vi "Dashboard Main.vi"() -> ()   [LabVIEW 2017]
uses:
  <vilib>/Utility/miscctls.llb/LVRowAndColumnTypeDef.ctl
  <vilib>/event_ctls.llb/eventvkey.ctl
  <vilib>/Rock Robotics/Network Tables/NT Read Numeric Array.vi
  <vilib>/Rock Robotics/Network Tables/NT Read Boolean.vi
  <vilib>/Rock Robotics/WPI/Dashboard/WPI_DashboardLogging Global.vi
panel:
  in  "Camera Settings Right":T1={"Frame Rate"=30, "Compression"=30, "Size"=1, "DB Camera Config"=FALSE} {"Frame Rate" scale=1.0..30.0; "Compression" scale=100.0..-1.0; "Size" items=["640x480", "320x240", "160x120"]}
  in  "Camera Name Right":string(combo)="No Camera Selection"
  out "Camera Info":cluster{"Mbps LED":bool, "Mbps":dbl, "fps":dbl} {"fps" format="%#.1g"; "Mbps" format="%#.1g"}
  in  "Camera Settings":T1={"Frame Rate"=30, "Compression"=30, "Size"=1, "DB Camera Config"=FALSE} {"Frame Rate" scale=1.0..30.0; "Compression" scale=100.0..-1.0; "Size" items=["640x480", "320x240", "160x120"]}
  in  "TCP":refnum<k5>
  in  "Rec Mode":enum32{"Stop", "Record", "Playback"}(radio)
  out "Robot IP":string
  out "Image Message":string="Timeout in Camera Communications"
  in  "Dashboard Tab":T2(tab)
  in  "Select Auto":string(combo)="Select Autonomous ..."
  out "NT Connection":bool
  out "MotorChart R":cluster{"Numeric":dbl, "Numeric":dbl}(graph)
  out "MotorChart L":cluster{"Numeric":dbl, "Numeric":dbl}(graph)
  out "MotorSliders R":cluster{"MotorSlide1":dbl, "MotorSlide2":dbl} {"MotorSlide2" scale=-1.0..1.0 scale format="%#_2e"; "MotorSlide1" scale=-1.0..1.0 scale format="%#_2e"}
  out "MotorSliders L":cluster{"MotorSlide1":dbl, "MotorSlide2":dbl} {"MotorSlide2" scale=-1.0..1.0 scale format="%#_2e"; "MotorSlide1" scale=-1.0..1.0 scale format="%#_2e"}
  out "Gyro":dbl(knob) scale=0.0..360.0
  out "JS1 Z":dbl(slide) scale=-1.0..1.0 scale format="%#_2e"
  out "JS1 Graph":cluster{"X":dbl, "Y":dbl}[](graph)
  out "JS1 Buttons":T3
  out "JS2 Z":dbl(slide) scale=-1.0..1.0 scale format="%#_2e"
  out "JS2 Graph":cluster{"X":dbl, "Y":dbl}[](graph)
  out "JS2 Buttons":T3
  out "Mode":T4(ring)=enum."Auto Disabled"
  out "Camera Image Right":T5(plugin-control)
  in  "DB/String 9":string
  in  "DB/String 8":string
  in  "DB/String 7":string
  in  "DB/String 6":string
  in  "DB/String 5":string
  in  "DB/String 4":string
  in  "DB/String 3":string
  in  "DB/String 2":string
  in  "DB/String 1":string
  in  "DB/String 0":string
  in  "DB/Slider 0":dbl(slide) scale=0.0..5.0
  in  "DB/Slider 1":dbl(slide) scale=0.0..5.0
  in  "DB/Slider 2":dbl(slide) scale=0.0..5.0
  in  "DB/Slider 3":dbl(slide) scale=0.0..5.0
  out "DB/LED 3":bool
  out "DB/LED 2":bool
  out "DB/LED 1":bool
  out "DB/LED 0":bool
  in  "DB/Button 3":bool
  in  "DB/Button 2":bool
  in  "DB/Button 1":bool
  in  "DB/Button 0":bool caption="New Name"
  out "Claw Right":bool
  out "Claw Left":bool
  out "Elevator Top":bool
  out "Elevator Bottom":bool
  out "Collector Limit Switch":bool
  out "fast":bool
  out "slow":bool
  out "Phase Indicator":string
  in  "Programming Level":dbl(knob) scale=0.0..11.0
  in  "What color are you?":string(combo)
  out "R3":u32(colorbox)
  out "R2":u32(colorbox)
  out "R1":u32(colorbox)
  out "L3":u32(colorbox)
  out "L2":u32(colorbox)
  out "L1":u32(colorbox)
  in  "Test Slider":dbl(slide) scale=0.0..100.0 scale format="%#_3g"
  in  "On/Off":bool caption="Solenoid"
  in  "Test Name":u16(ring) items=["Select the test to run..."]
  in  "Test Tree":string(tree)
  in  "Motor":cluster{"Value":dbl, "Enable":bool} {"Value" scale=-1.0..1.0 scale format="%#_3g"}
  out "Progress":T6 {"Test Progress" scale=0.0..100.0}
  in  "Rev/Fwd":cluster{"Forward":bool, "Reverse":bool}
  in  "Test Ring":u16(ring) items=["Monochrome", "Color"]
  out "Cmd Status":string
  in  "Execute Command":bool
  in  "Command Params":string[][](table)
  in  "Command Selection":i32(listbox)
  in  "CheckList":i32(listbox)
  out "Tree":string(tree)
  out "Camera Image":T5(plugin-control)
  out "Background":bool
  in  "Camera Name":string(combo)="No Camera Selection"
  # "HW"
  # "HW"
  # "Joysticks"
  # "Drive Motors"
  # "Front"
  # "Right"
  # "Left"
  # "Back"
  # "If you need that extra push over the cliff put it to eleven. These go to eleven."
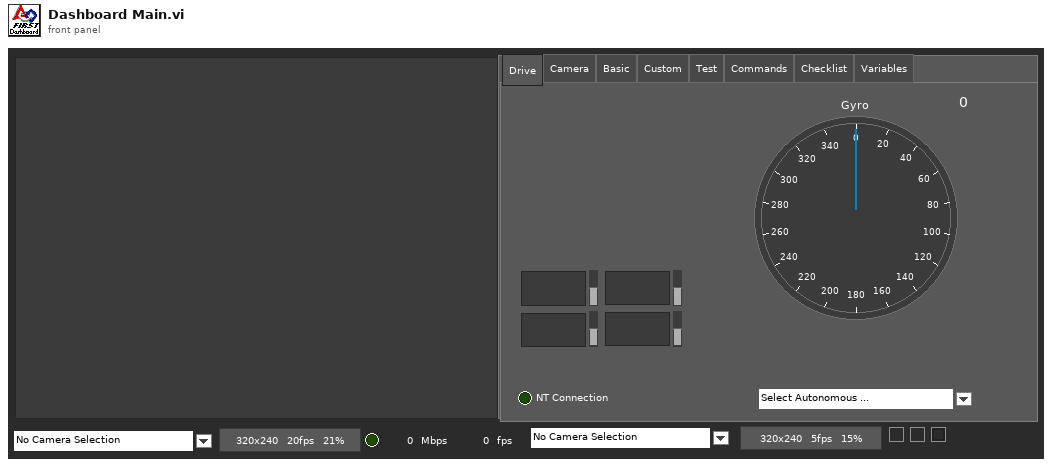
[diagram p1: front panel]
types:
  T1 = cluster{"Frame Rate":i32, "Compression":i32, "Size":u16, "DB Camera Config":bool}
  T2 = enum32{"Drive", "Camera", "Basic", "Custom", "Test", "Commands", "Checklist", "Variables"}
  T3 = cluster{bool, bool, bool, bool, bool, bool, bool, bool, bool, bool, bool, bool}
  T4 = enum8{"Tele-Op Disabled", "Tele-Op Enabled", "Auto Disabled", "Auto Enabled", "Test Disabled", "Test Enabled", "Disconnected", "No Code", "E-Stop"}
  T5 = typedef "IMAQ Image.ctl" = refnum<image>
  T6 = cluster{"Test Progress":u8, "Test Progress Text":string}
  T7 = cluster{"Save Path":path, "Interval (s)":dbl, "Keep":i32}
  T8 = typedef "Image Type" = u32
  T9 = cluster{"IDs":cluster{"RPC field ID":u16, "Unique ID":u16}, "String":string}
  T10 = cluster{"Error Strings":string, "Disable Counts":cluster{u16, u16}, "Rail Faults":cluster{u16, u16, u16}, "Robot IP":string, "DB Mode":u8, "Event Info":cluster{"Name":string, "Type":u8, "Number":u16, "Replay":u8}}
  T11 = cluster{"Storage":cluster{"Disk Free":u64, "RAM Block":u32, "RAM free":u32}, "CPU Utilization":cluster{"CPU % ISR":sgl, "CPU % Time Crit":sgl, "CPU % Timed Str":sgl, "CPU % High":sgl, "CPU % Above":sgl, "CPU % Normal":sgl, "CPU % Low":sgl}, "CAN":cluster{"% Bus Utilization":sgl, "Bus Off Cnt":u32, "TX_FIFO Full Cnt":u32, "Receive Error Cnt":u8, "Transmit Error Cnt":u8}, "HID":cluster{"HID Outputs":u32, "Rumble Low":u16, "Rumble High":u16}[]}
  T12 = cluster{"Status bits":cluster{"Test Mode":bool, "Autonomous":bool, "Enabled":bool, "Code Start":bool, "Brownout":bool, "Reserved 2":bool, "Reserved 3":bool, "E-Stop":bool}, "Code Trace":cluster{"Disabled":bool, "TeleOp":bool, "Auto":bool, "Test":bool}, "Controller Type":enum16{"unknown", "cRIO", "roboRio"}, "Code?":enum16{"unknown", "noCode", "code"}, "Battery V":dbl}
  T13 = cluster{"Control Bits":cluster{"TestMode":bool, "Autonomous":bool, "Enabled":bool, "FMS Present":bool, bool, bool, bool, "E-Stop":bool}, "Team Station ":u8, "Countdown":sgl, "Joystick Values":cluster{"Axes":dbl[], "Buttons":bool[], "POVs":i16[]}[]}
  T14 = cluster{"Axes":dbl[], "Buttons":bool[], "POVs":i16[]}[]
  T15 = cluster{"Axes":dbl[], "Buttons":bool[], "POVs":i16[]}
  T16 = cluster{"Buttons[0]":bool, "Buttons[1]":bool, "Buttons[2]":bool, "Buttons[3]":bool, "Buttons[4]":bool, "Buttons[5]":bool, "Buttons[6]":bool, "Buttons[7]":bool, "Buttons[8]":bool, "Buttons[9]":bool, "Buttons[10]":bool, "Buttons[11]":bool}
  T17 = cluster{"Camera Image":refnum<vi>, "Dashboard Tab":refnum<vi>, "Background":refnum<vi>, "Rec Mode":refnum<vi>, "Test Slider":refnum<vi>, "On/Off ":refnum<vi>, "Test Ring":refnum<vi>, "Rev/Fwd":refnum<vi>, "Test Name":refnum<vi>, "Motor":refnum<vi>, "Progress":refnum<vi>, "CheckList":refnum<vi>, "Tree":refnum<vi>, "Test Tree":refnum<vi>, "Command Params":refnum<vi>, "Command Selection":refnum<vi>, "Execute Command":refnum<vi>, "Cmd Status":refnum<vi>, "Camera Settings":refnum<vi>, "Camera Name":refnum<vi>, "Camera Info":refnum<vi>, "Camera Settings Right":refnum<vi>, "Camera Name Right":refnum<vi>, "Camera Image Right":refnum<vi>}
  T18 = cluster{"Camera Name":string, string, "Saved DB Images Info":cluster{"Save Path":path, "Interval (s)":dbl, "Keep":i32}}
  T19 = cluster{"Camera Name Right":string, string, "Saved DB Images Info":cluster{"Save Path":path, "Interval (s)":dbl, "Keep":i32}}
  T20 = cluster{"Operation":enum16{"Update", "Clear"}, "Color Box":u32}[]
  T21 = typedef "eventvkey.ctl" = enum16{"ASCII", "Enter", "Return", "Shift", "Ctrl", "Alt", "Cmd", "Opt", "Caps", "NumLock", "Clear", "Break", "Up", "Down", "Left", "Right", "Insert", "Delete", "Home", "End", "PageUp", "PageDown", "Escape", "Help", "Pause", "ScrollLock", "F1", "F2", "F3", "F4", "F5", "F6", "F7", "F8", "F9", "F10", "F11", "F12", "F13", "F14", "F15", "F16", "F17", "F18", "F19", "F20", "F21", "F22", "F23", "F24", "Play", "VolumeUp", "VolumeDown", "Mute", "Two Byte Char"}
  T22 = cluster{"Image Size":bool, "Image Type":bool, "Pixel Value":bool, "ROI Information":bool, "Zoom Factor":bool}
  T23 = cluster{"Operation":enum16{"Update", "Clear"}, "Color Box":u32}
  T24 = typedef "LVRowAndColumnTypeDef.ctl" = cluster{"Row":i32, "Column":i32}
  T25 = cluster{"Shift":bool, "Ctrl":bool, "Alt":bool, "Cmd":bool, "Opt":bool}
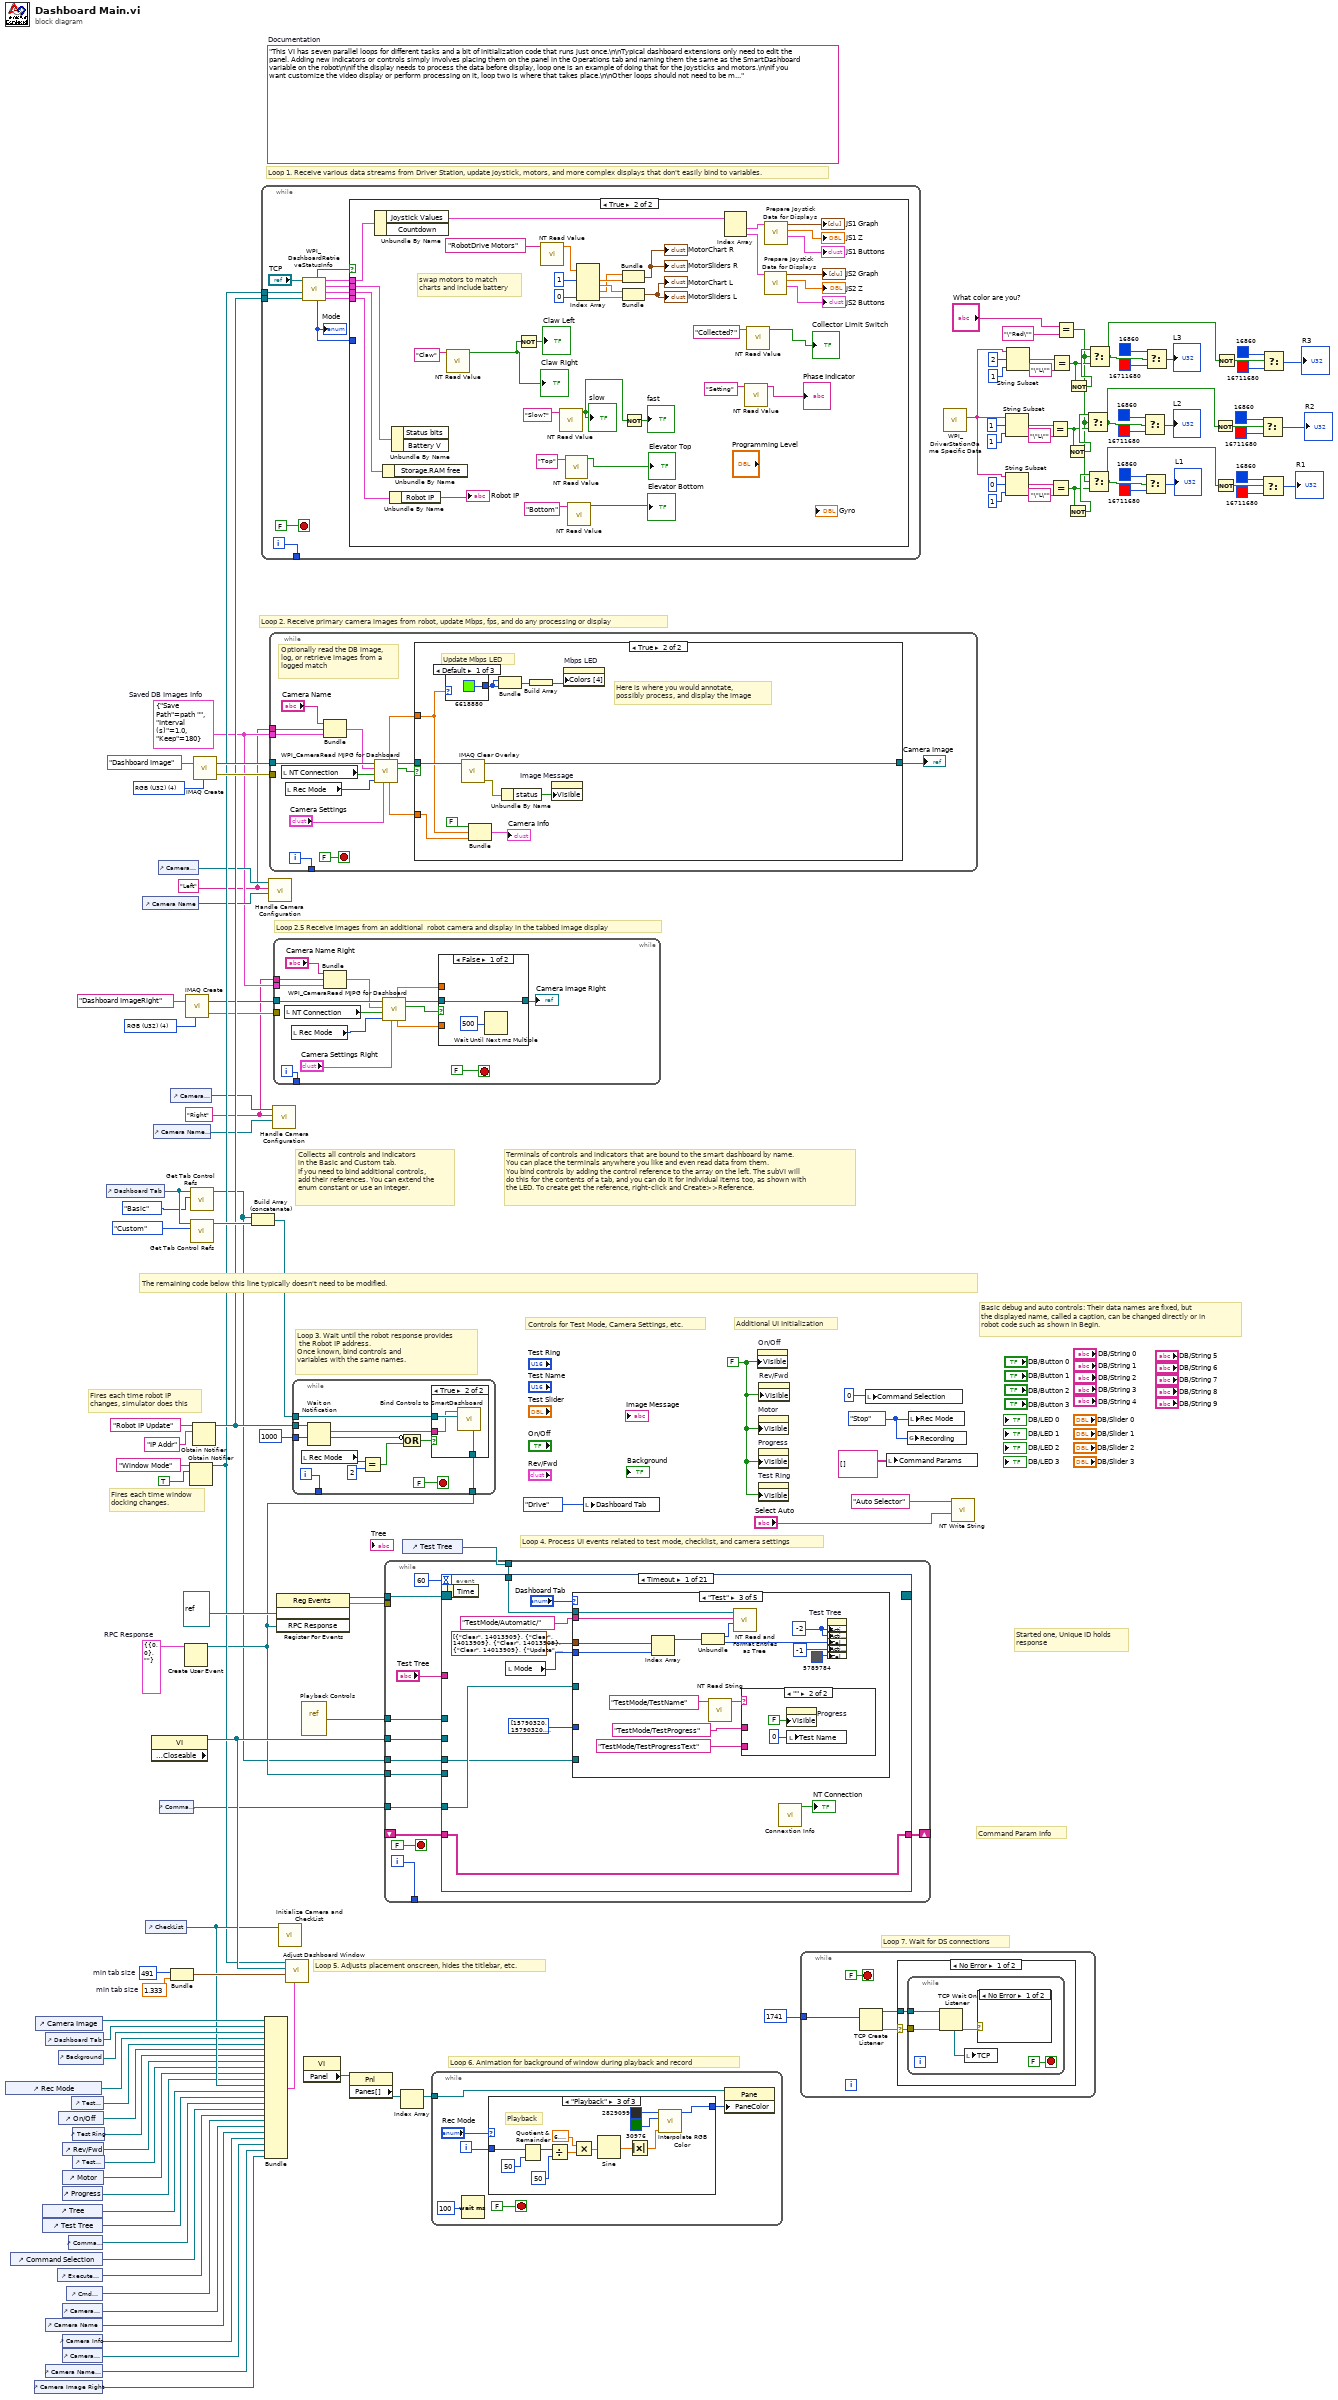
[diagram p0: block diagram]
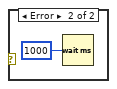
[diagram p3: hidden frame]
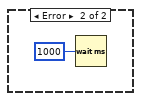
[diagram p4: hidden frame]
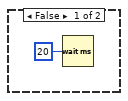
[diagram p5: hidden frame]
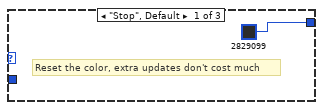
[diagram p6: hidden frame]
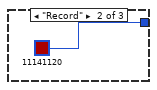
[diagram p7: hidden frame]
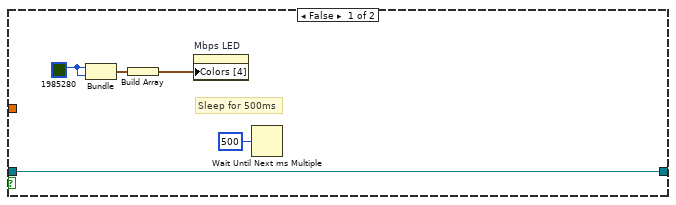
[diagram p9: hidden frame]
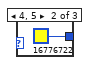
[diagram p10: hidden frame]
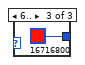
[diagram p11: hidden frame]
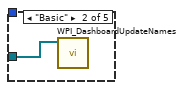
[diagram p13: hidden frame]
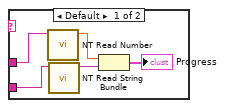
[diagram p14: hidden frame]
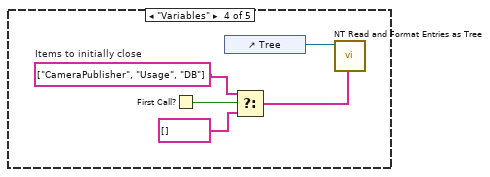
[diagram p15: hidden frame]
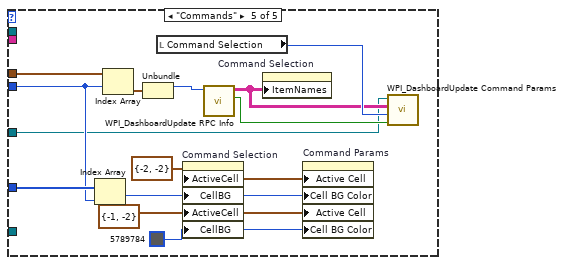
[diagram p16: hidden frame]
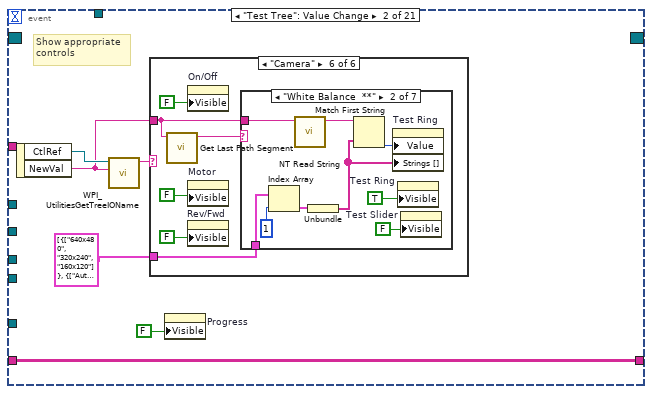
[diagram p17: hidden frame]
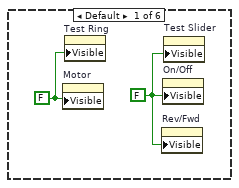
[diagram p18: hidden frame]
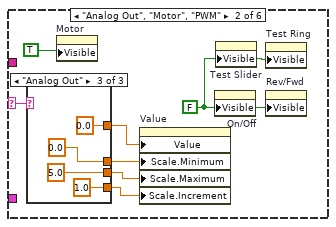
[diagram p19: hidden frame]
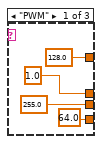
[diagram p20: hidden frame]
diagram:
  w49 = T7 {"Save Path"=path "", "Interval (s)"=1.0, "Keep"=180}  # Saved DB Images Info
  w48 = "Right"
  w47 = "Left"
  w59 = T8 4 items=["Grayscale (U8)", "Grayscale (I16)", "Grayscale (SGL)", "Complex (CSG)", "RGB (U32)", "HSL (U32)", "RGB (U64)"] ("Image Type")
  w75 = T9 {"IDs"={"RPC field ID"=0, "Unique ID"=0}, "String"=""}  # RPC Response
  w98 = 491  # min tab size
  w97 = 1.333  # min tab size
  w105 = enum32{"Stop", "Record", "Playback"}."Stop" ("Rec Mode")
  w82 = FALSE ("Visible")
  (unwired) "This VI has seven parallel loops for different tasks and a bit of initialization code that runs just once.\n\nTypical dashboard extensions only need to edit the panel. Adding new indicators or controls simply involves placing them on the panel in the Operations tab and naming them the same as the SmartDashboard variable on the robot\n\nIf the display needs to process the data before display, loop one is an example of doing that for the joysticks and motors.\n\nIf you want customize the video display or perform processing on it, loop two is where that takes place.\n\nOther loops should not need to be modified. They are pretty standard, and document the task they perform."  # Documentation
  w122 = T8 4 items=["Grayscale (U8)", "Grayscale (I16)", "Grayscale (SGL)", "Complex (CSG)", "RGB (U32)", "HSL (U32)", "RGB (U64)"] ("Image Type")
  # "Loop 2.5 Receive images from an additional  robot camera and display in the tabbed image display"
  # "Command Param Info"
  # "Started one, Unique ID holds\nresponse"
  # "Loop 7. Wait for DS connections"
  # "Basic debug and auto controls: Their data names are fixed, but\nthe displayed name, called a caption, can be changed directly or in\nrobot code such as shown in Begin."
  # "Controls for Test Mode, Camera Settings, etc."
  # "Additional UI Initialization"
  # "Loop 6. Animation for background of window during playback and record"
  # "Fires each time robot IP\nchanges, simulator does this"
  # "Fires each time window\ndocking changes."
  # "Collects all controls and indicators\nin the Basic and Custom tab.\nIf you need to bind additional controls,\nadd their references. You can extend the\nenum constant or use an integer."
  # "The remaining code below this line typically doesn't need to be modified."
  # "Loop 4. Process UI events related to test mode, checklist, and camera settings"
  # "Terminals of controls and indicators that are bound to the smart dashboard by name.\nYou can place the terminals anywhere you like and even read data from them.\nYou bind controls by adding the control reference to the array on the left. The subVI will\ndo this for the contents of a tab, and you can do it for individual items too, as shown with\nthe LED. To create get the reference, right-click and Create>>Reference."
  # "Loop 3. Wait until the robot response provides\n the Robot IP address.\nOnce known, bind controls and\nvariables with the same names."
  # "Loop 5. Adjusts placement onscreen, hides the titlebar, etc."
  # "Loop 1. Receive various data streams from Driver Station, update joystick, motors, and more complex displays that don't easily bind to variables."
  # "Loop 2. Receive primary camera images from robot, update Mbps, fps, and do any processing or display"
  n1 = control-ref of="Rec Mode"() -> (w88:refnum<vi>)
  n2 = control-ref of="Command Selection"() -> (w74:refnum<vi>)
  n3 = control-ref of="Camera Image Right"() -> (w52:refnum<vi>)
  n4 = control-ref of="Camera Image"() -> (w100:refnum<vi>)
  n5 = control-ref of="Tree"() -> (w92:refnum<vi>)
  n6 = control-ref of="Test Tree"() -> (w91:refnum<vi>)
  n7 = control-ref of="Dashboard Tab"() -> (w99:refnum<vi>)
  n8 = control-ref of="Camera Name"() -> (w65:refnum<vi>)
  n9 = control-ref of="Camera Name Right"() -> (w53:refnum<vi>)
  n10 = control-ref of="Execute Command"() -> (w76:refnum<vi>)
  n11 = control-ref of="Background"() -> (w95:refnum<vi>)
  n12 = control-ref of="On/Off"() -> (w86:refnum<vi>)
  n13 = control-ref of="Progress"() -> (w83:refnum<vi>)
  n14 = control-ref of="Camera Settings"() -> (w66:refnum<vi>)
  n15 = control-ref of="Camera Info"() -> (w64:refnum<vi>)
  n16 = control-ref of="Camera Settings Right"() -> (w54:refnum<vi>)
  n17 = control-ref of="Rev/Fwd"() -> (w84:refnum<vi>)
  n18 = control-ref of="Motor"() -> (w89:refnum<vi>)
  n19 = control-ref of="Cmd Status"() -> (w70:refnum<vi>)
  n20 = control-ref of="Command Params"() -> (w77:refnum<vi>)
  n21 = control-ref of="Test Slider"() -> (w87:refnum<vi>)
  n22 = control-ref of="Test Ring"() -> (w85:refnum<vi>)
  n23 = control-ref of="Test Name"() -> (w90:refnum<vi>)
  n24 = control-ref of="Dashboard Tab"() -> (w103:refnum<vi>)
  n25 = control-ref of="Camera Name"() -> (w67:refnum<vi>)
  n26 = control-ref of="CheckList"() -> (w93:refnum<vi>)
  n27 = property class="VI" props=["Front Panel.Closeable"]() -> (reference out=w104:refnum<vi>)  [unwired: 2 in, 2 out]
  n28 = control-ref of="Camera Name Right"() -> (w55:refnum<vi>)
  n29 = control-ref of="Camera Settings"() -> (w68:refnum<vi>)
  n30 = control-ref of="Command Params"() -> (w69:refnum<vi>)
  n31 = control-ref of="Camera Settings Right"() -> (w56:refnum<vi>)
  n32 = Bundle("min tab size"=w98, "min tab size"=w97) -> (w96:cluster{"min tab size":i32, "min tab size":dbl})  [unwired: 1 in]
  n33 = Create User Event(user event datatype=w75) -> (user event=w71:refnum<user-event>)  [unwired: 1 in, 1 out]
  n34 = call "IMAQ Create"("Image Name"="Dashboard ImageRight", "Image Type"=w59) -> ("New Image"=w58:T5, "error out"=w57:errorcluster)  [unwired: 2 in, 1 out]
  n35 = Obtain Notifier(name (unnamed)="Window Mode", notification data type=TRUE) -> (notifier out=w80:refnum<notifier>)  [unwired: 2 in, 2 out]
  n36 = call <vilib>:"Get Tab Control Refs.vi"("Page Index"=T2."Basic" ("Dashboard Tab"), "TabControl in"=w103) -> ("ControlsOnPage"=w63:refnum<vi>[])  [unwired: 9 in]
  n37 = call <vilib>:"Get Tab Control Refs.vi"("Page Index"=T2."Custom" ("Dashboard Tab"), "TabControl in"=w103) -> ("ControlsOnPage"=w102:refnum<vi>[])  [unwired: 9 in]
  n38 = Obtain Notifier(name (unnamed)="Robot IP Update", notification data type="IP Addr" ("name (unnamed)")) -> (notifier out=w81:refnum<notifier>)  [unwired: 2 in, 2 out]
  n39 = call "IMAQ Create"("Image Name"="Dashboard Image", "Image Type"=w122) -> ("New Image"=w120:T5, "error out"=w119:errorcluster)  [unwired: 2 in, 1 out]
  n40 = Build Array (concatenate)(w63, w102) -> (w101:refnum<vi>[])
  n41 = while {
    tunnel: [w132] -> _
    tunnel: w81 -> [w126]
    tunnel: w80 -> [w123]
    i -> [w132]
    stop <- FALSE stop-if-true
    n42 = call <vilib>:"WPI_DashboardRetrieveStatusInfo.vi"("Binding Refnum"=w126, "Window Mode Notifier"=w123, "TCP Cnx"="TCP") -> ("Power and Errors"=w127:T10, "Robot Metrics"=w130:T11, "Status Info"=w131:T12, "Control Info"=w128:T13, "Robot Mode"=w125:T4, "Process?"=w129:bool)  [unwired: 3 in]
    "Mode" <- w125
    n43 = case shown="True" w129 {
      tunnel: w131 -> [_ w172]
      tunnel: w130 -> [_ w171]
      tunnel: w128 -> [_ w170]
      tunnel: w127 -> [_ w169]
      tunnel: w125 -> [_ _]
      frame False {
        n44 = Wait (ms)(milliseconds to wait=u32 20) -> ()  [unwired: 1 out]
      }
      frame True {
        # "swap motors to match\ncharts and include battery"
        n45 = Unbundle By Name(w170) -> ("Joystick Values"=w160:T14)  [unwired: 1 out]
        n46 = Unbundle By Name(w171) -> ()  [unwired: 1 out]
        n47 = Unbundle By Name(w169) -> ("Robot IP"=→"Robot IP":string)
        n48 = Unbundle By Name(w172) -> ()  [unwired: 2 out]
        n49 = call-poly <vilib>:"NT Read Value.vi"("Name"="Claw") -> ("Boolean"=w135:bool)  [unwired: 9 in, 1 out]
        "Claw Right" <- w135
        n50 = Not(x=w135) -> (.not. x?=→"Claw Left":bool)
        n51 = call-poly <vilib>:"NT Read Value.vi"("Name"="RobotDrive Motors") -> ("Numeric Array"=w150:dbl[])  [unwired: 9 in, 1 out]
        n52 = call-poly <vilib>:"NT Read Value.vi"("Name"="Slow?") -> ("Boolean"=w143:bool)  [unwired: 9 in, 1 out]
        "slow" <- w143
        n53 = call-poly <vilib>:"NT Read Value.vi"("Name"="Top") -> ("Boolean"=→"Elevator Top":bool)  [unwired: 9 in, 1 out]
        n54 = call-poly <vilib>:"NT Read Value.vi"("Name"="Bottom") -> ("Boolean"=→"Elevator Bottom":bool)  [unwired: 9 in, 1 out]
        n55 = Index Array(array=w150, index #1=1, index #4=0) -> (element #1=w164:dbl, element #2=w165:dbl, element #3=w163:dbl, element #4=w168:dbl)  [unwired: 2 in]
        n56 = Bundle("Numeric"=w163, "Numeric"=w164) -> (→"MotorChart R" →"MotorSliders R":cluster{"Numeric":dbl, "Numeric":dbl})  [unwired: 1 in]
        n57 = Bundle("Numeric"=w165, "Numeric"=w168) -> (→"MotorChart L" →"MotorSliders L":cluster{"Numeric":dbl, "Numeric":dbl})  [unwired: 1 in]
        n58 = Not(x=w143) -> (.not. x?=→"fast":bool)
        n59 = Index Array(array=w160) -> (element #1=w159:T15, element #2=w155:T15)  [unwired: 2 in]
        n60 = call-poly <vilib>:"NT Read Value.vi"("Name"="Setting") -> ("String"=→"Phase Indicator":string)  [unwired: 9 in, 1 out]
        n61 = call-poly <vilib>:"NT Read Value.vi"("Name"="Collected?") -> ("Boolean"=→"Collector Limit Switch":bool)  [unwired: 9 in, 1 out]
        n62 = call "Prepare Joystick Data for Displays.vi"("Joystick Values"=w155) -> ("Buttons"=→"JS2 Buttons":T16, "Z Axis"=→"JS2 Z":dbl, "Cartesian Data"=→"JS2 Graph":cluster{"X axis":dbl, "X axis":dbl}[])  [unwired: 8 in]
        n63 = call "Prepare Joystick Data for Displays.vi"("Joystick Values"=w159) -> ("Buttons"=→"JS1 Buttons":T16, "Z Axis"=→"JS1 Z":dbl, "Cartesian Data"=→"JS1 Graph":cluster{"X axis":dbl, "X axis":dbl}[])  [unwired: 8 in]
      }
    }
  }
  n64 = Bundle("Camera Image"=w100, "Dashboard Tab"=w99, "Background"=w95, "Rec Mode"=w88, "Test Slider"=w87, "On/Off"=w86, "Test Ring"=w85, "Rev/Fwd"=w84, "Test Name"=w90, "Motor"=w89, "Progress"=w83, "CheckList"=w93, "Tree"=w92, "Test Tree"=w91, "Command Params"=w77, "Command Selection"=w74, "Execute Command"=w76, "Cmd Status"=w70, "Camera Settings"=w66, "Camera Name"=w65, "Camera Info"=w64, "Camera Settings Right"=w54, "Camera Name Right"=w53, "Camera Image Right"=w52) -> (w94:T17)  [unwired: 1 in]
  n65 = call "Handle Camera Configuration.vi"("CameraNameRef"=w67, "Display Name"=w47, "ClusterRef"=w68) -> ()  [unwired: 9 in]
  n66 = while {
    tunnel: w120 -> [w185]
    tunnel: w119 -> [_]
    tunnel: [w186] -> _
    tunnel: w49 -> [w176]
    tunnel: w47 -> [w173]
    i -> [w186]
    stop <- FALSE stop-if-true
    # "Optionally read the DB image,\nlog, or retrieve images from a\nlogged match"
    n67 = local read "NT Connection"() -> (w177:bool)
    n68 = local read "Rec Mode"() -> (w181:enum32{"Stop", "Record", "Playback"})
    n69 = Bundle("Camera Name"="Camera Name", w173, "Saved DB Images Info"=w176) -> (w175:T18)  [unwired: 1 in]
    n70 = call <vilib>:"WPI_CameraRead MJPG for Dashboard.vi"("Camera Settings"="Camera Settings", "Rec Mode"=w181, "NT Connection"=w177, "Capture Info"=w175, "Refnum in"=w185) -> ("Active"=w183:bool, "Refnum out"=w184:T5, "FPS"=w182:dbl, "Bandwidth (Mbps)"=w180:dbl)  [unwired: 3 in]
    n71 = case shown="True" w183 {
      tunnel: w184 -> [w188 w199]
      tunnel: w180 -> [_ w196]
      tunnel: w182 -> [_ w197]
      tunnel: [w188 w193] -> w178
      frame False {
        w190 = u32 1985280 ("Color Box")
        # "Sleep for 500ms"
        n72 = Bundle("Color Box"=w190, "Color Box"=w190) -> (w191:cluster{"Color Box":u32, "Color Box":u32})  [unwired: 1 out]
        n73 = Build Array(w191) -> (w189:cluster{"Color Box":u32, "Color Box":u32}[])
        n74 = property on="Mbps LED" class="Bool (strict)"("Colors [4]"=w189) -> ()  [unwired: 2 in, 2 out]
        n75 = Wait Until Next ms Multiple(millisecond multiple=u32 500) -> ()  [unwired: 1 out]
      }
      frame True {
        # "Here is where you would annotate,\npossibly process, and display the image"
        # "Update Mbps LED"
        n76 = case shown="Default" w196 {
          tunnel: [u32 6618880 ("Color Box") u32 16776722 ("Color Box") u32 16716800 ("Color Box")] -> w200
          frame Default {
          }
          frame 4, 5 {
          }
          frame 6.. {
          }
        }
        n77 = call "IMAQ Clear Overlay"("Image"=w199) -> ("error out"=w202:errorcluster, "Image Out"=w193:T5)  [unwired: 2 in, 7 out]
        n78 = Bundle(FALSE, "Bandwidth (Mbps)"=w196, "FPS"=w197) -> (→"Camera Info":cluster{bool, "Bandwidth (Mbps)":dbl, "FPS":dbl})  [unwired: 1 in]
        n79 = Bundle("Color Box"=w200, "Color Box"=w200) -> (w201:cluster{"Color Box":u32, "Color Box":u32})  [unwired: 1 out]
        n80 = Unbundle By Name(w202) -> ("status"=w203:bool)
        n81 = Build Array(w201) -> (w198:cluster{"Color Box":u32, "Color Box":u32}[])
        n82 = property on="Image Message" class="Str"("Visible"=w203) -> ()  [unwired: 2 in, 2 out]
        n83 = property on="Mbps LED" class="Bool (strict)"("Colors [4]"=w198) -> ()  [unwired: 2 in, 2 out]
      }
    }
    "Camera Image" <- w178
  }
  n84 = call "Handle Camera Configuration.vi"("CameraNameRef"=w55, "Display Name"=w48, "ClusterRef"=w56) -> ()  [unwired: 9 in]
  n85 = while {
    tunnel: w58 -> [w221]
    tunnel: w57 -> [_]
    tunnel: [w216] -> _
    tunnel: w49 -> [w210]
    tunnel: w48 -> [w207]
    i -> [w216]
    stop <- FALSE stop-if-true
    n86 = local read "NT Connection"() -> (w211:bool)
    n87 = local read "Rec Mode"() -> (w220:enum32{"Stop", "Record", "Playback"})
    n88 = Bundle("Camera Name Right"="Camera Name Right", w207, "Saved DB Images Info"=w210) -> (w209:T19)  [unwired: 1 in]
    n89 = call <vilib>:"WPI_CameraRead MJPG for Dashboard.vi"("Camera Settings"="Camera Settings Right", "Rec Mode"=w220, "NT Connection"=w211, "Capture Info"=w209, "Refnum in"=w221) -> ("Active"=w215:bool, "Refnum out"=w218:T5, "FPS"=w213:dbl, "Bandwidth (Mbps)"=w214:dbl)  [unwired: 3 in]
    n90 = case shown="False" w215 {
      tunnel: w218 -> [w222 w224]
      tunnel: w214 -> [_ _]
      tunnel: w213 -> [_ _]
      tunnel: [w222 w224] -> w212
      frame False {
        n91 = Wait Until Next ms Multiple(millisecond multiple=u32 500) -> ()  [unwired: 1 out]
      }
      frame True {
      }
    }
    "Camera Image Right" <- w212
  }
  n92 = register-events(refnum<vi> refnum, w71) -> (reference out=w109:refnum<event-registration>, error out=w108:errorcluster)  [unwired: 2 in]
  n93 = call "Initialize Camera and CheckList.vi"("ListBox in"=w93) -> ()  [unwired: 11 in]
  n94 = call "Adjust Dashboard Window.vi"("Sizing Refnums"=w94, "Size Constraints"=w96, "VI"=w104, "WIn Mode"=w80) -> ()  [unwired: 8 in]
  n95 = while {
    tunnel: w101 -> [w236]
    tunnel: w81 -> [w234]
    tunnel: [w232] -> _
    tunnel: u32 1000 ("milliseconds to wait") -> [w231]
    tunnel: w71 -> [w225]
    i -> [w232]
    stop <- FALSE stop-if-true
    n96 = local read "Rec Mode"() -> (w227:enum32{"Stop", "Record", "Playback"})
    n97 = Wait on Notification(notifier=w234, timeout in ms (-1)=w231) -> (notification=w233:string, timed out?=w229:bool)  [unwired: 2 in, 2 out]
    n98 = Equal?(x=w227, y=u16 2 ("Rec Mode")) -> (x = y?=w228:bool)
    n99 = Compound Arithmetic op=OR(invert w229, w228) -> (w230:bool)
    n100 = case shown="True" w230 {
      tunnel: w236 -> [_ w239]
      tunnel: w233 -> [_ w238]
      tunnel: w225 -> [_ w237]
      frame False {
      }
      frame True {
        n101 = call <vilib>:"Bind Controls to SmartDashboard.vi"("RPC ref"=w237, "Bound Control Refs"=w239, "Server IP Address"=w238) -> ()  [unwired: 9 in]
      }
    }
  }
  n102 = vi-ref "Playback Controls.vi"() -> (w110:refnum<vi>)
  n103 = property class="VI"() -> ("Panel"=w112:refnum<vi>)  [unwired: 2 in, 2 out]
  n104 = property class="Pnl"(reference=w112) -> ("Panes[]"=w113:refnum<vi>[])  [unwired: 1 in, 2 out]
  n105 = Index Array(array=w113) -> (element=w111:refnum<vi>)  [unwired: 1 in]
  n106 = control-ref of="Test Tree"() -> (w114:refnum<vi>)
  n107 = while {
    tunnel: [w249] -> _
    tunnel: w114 -> [w248]
    tunnel: w110 -> [w247]
    tunnel: w109 -> [w246]
    tunnel: w108 -> [_]
    tunnel: w104 -> [w245]
    tunnel: w71 -> [w244]
    tunnel: w69 -> [w243]
    shift-right: [w242] -> _
    shift-left: _ -> [w241]
    tunnel: w63 -> [w240]
    i -> [w249]
    stop <- FALSE stop-if-true
    n108 = event shown="[0] Timeout" {
      selector: w246 -> [_ _ _ _ _ _ _ _ _ _ _ _ _ _ _ _ _ _ _ _ _]
      dyn-events: [_ _ _ _ _ _ _ _ _ _ _ _ _ _ _ _ w509 _ _ _ _] -> _
      timeout: u32 60 ("milliseconds to wait") -> [_ _ _ _ _ _ _ _ _ _ _ _ _ _ _ _ _ _ _ _ _]
      tunnel: w248 -> [w261 _ _ _ _ _ _ _ _ _ _ _ _ _ _ _ _ _ _ _ _]
      tunnel: "Test Tree" -> [_ _ _ _ _ _ _ _ _ _ _ w476 w484 w486 w490 w498 _ _ _ _ _]
      tunnel: w247 -> [_ _ _ _ _ _ _ _ _ _ _ _ _ _ _ _ w511 _ w529 _ _]
      tunnel: w245 -> [_ _ _ _ _ _ _ _ _ _ _ _ _ _ _ _ w507 _ _ _ _]
      tunnel: w244 -> [_ _ _ _ _ _ _ _ _ _ _ _ _ _ _ _ w505 _ _ _ _]
      tunnel: w243 -> [w256 _ _ _ _ _ w427 _ _ _ _ _ _ _ _ _ _ _ _ _ _]
      tunnel: [w255 w304 w406 w411 w420 w424 w425 w434 w444 w451 w463 w475 w482 w485 w489 w497 w504 w524 w526 w530 w543] -> w242
      tunnel: w241 -> [w255 w304 w406 w411 w420 w424 w425 _ _ w451 w463 w475 w482 w485 w489 w497 w504 w524 w526 w530 w543]
      tunnel: w240 -> [w253 _ _ _ _ _ _ _ _ _ _ _ _ _ _ _ _ _ _ _ _]
      event Timeout {
        n109 = event-data() -> ()  [unwired: 1 in, 1 out]
        n110 = local read "Mode"() -> (w258:T4)
        n111 = case shown="\"Test\"" "Dashboard Tab" {
          tunnel: w261 -> [_ _ w277 _ _]
          tunnel: "TestMode/Automatic/" ("Name Pattern") -> [_ _ w276 _ _]
          tunnel: T20 [{"Operation"=enum."Clear", "Color Box"=14013909}, {"Operation"=enum."Clear", "Color Box"=14013909}, {"Operation"=enum."Clear", "Color Box"=14013909}, {"Operation"=enum."Clear", "Color Box"=14013909}, {"Operation"=enum."Update", "Color Box"=14013909}, {"Operation"=enum."Update", "Color Box"=16777215}, {"Operation"=enum."Clear", "Color Box"=14013909}, {"Operation"=enum."Clear", "Color Box"=14013909}, {"Operation"=enum."Clear", "Color Box"=14013909}] -> [_ _ w269 _ w297]
          tunnel: w258 -> [_ _ w268 _ w296]
          tunnel: u32[] [15790320, 15790320, 15790320, 15790320, 16777215, 16777215, 15790320, 15790320, 15790320] -> [_ _ _ _ w302]
          tunnel: w256 -> [_ _ _ _ w290]
          tunnel: w253 -> [_ w263 _ _ _]
          frame "Custom", Default {
          }
          frame "Basic" {
            n112 = call <vilib>:"WPI_DashboardUpdateNames.vi"("Controls on Tab"=w263) -> ()  [unwired: 11 in]
          }
          frame "Test" {
            w275 = -2 ("Active Item:Row Number")
            n113 = Index Array(array=w269, index=w268) -> (element=w270:T23)
            n114 = Unbundle(w270) -> ("Operation"=w271:enum16{"Update", "Clear"}, "Color Box"=w272:u32)
            n115 = call <vilib>:"NT Read String.vi"("Name"="TestMode/TestName") -> ("String"=w266:string)  [unwired: 9 in, 1 out]
            n116 = call <vilib>:"NT Read and Format Entries as Tree.vi"("Operation"=w271, "Name Pattern"=w276, "Tree Refnum"=w277) -> ()  [unwired: 7 in, 2 out]
            n117 = case shown="\"\"" w266 {
              tunnel: "TestMode/TestProgress" ("Name") -> [w279 _]
              tunnel: "TestMode/TestProgressText" ("Name") -> [w278 _]
              frame Default {
                n118 = call <vilib>:"NT Read Number.vi"("Name"=w279) -> ("Numeric"=w280:dbl)  [unwired: 9 in, 1 out]
                n119 = call <vilib>:"NT Read String.vi"("Name"=w278) -> ("String"=w281:string)  [unwired: 9 in, 1 out]
                n120 = Bundle("Numeric"=w280, "String"=w281) -> (→"Progress":cluster{"Numeric":dbl, "String":string})  [unwired: 1 in]
              }
              frame "" {
                n121 = property on="Progress" class="Clust (strict)"("Visible"=FALSE) -> ()  [unwired: 2 in, 2 out]
                n122 = local write "Test Name"(u16 0) -> ()
              }
            }
            n123 = property on="Test Tree" class="Tree (strict)"("Active Item Row Number"=w275, "ActiveColNum"=w275, "CellBG"=w272, "Active Item Row Number"=-1 ("Active Item:Row Number"), "CellBG"=u32 5789784 ("Color Box")) -> ()  [unwired: 2 in, 2 out]
          }
          frame "Variables" {
            w287 = string[] ["CameraPublisher", "Usage", "DB"]  # Items to initially close
            n124 = First Call?() -> (First Call?: T/F=w288:bool)
            n125 = control-ref of="Tree"() -> (w289:refnum<vi>)
            n126 = Select(t=w287, s=w288, f=string[] []) -> (s? t:f=w285:string[])
            n127 = call <vilib>:"NT Read and Format Entries as Tree.vi"("Tags to  Close"=w285, "Tree Refnum"=w289) -> ()  [unwired: 8 in, 2 out]
          }
          frame "Commands" {
            w298 = u32 5789784 ("Color Box")
            w299 = T24 {"Row"=-1, "Column"=-2} ("Active Cell:Active Cell")
            w301 = T24 {"Row"=-2, "Column"=-2} ("Active Cell:Active Cell")
            n128 = Index Array(array=w302, index=w296) -> (element=w300:u32)
            n129 = Index Array(array=w297, index=w296) -> (element=w295:T23)
            n130 = Unbundle(w295) -> ("Operation"=w294:enum16{"Update", "Clear"})  [unwired: 1 out]
            n131 = local read "Command Selection"() -> (w293:i32)
            n132 = property on="Command Selection" class="MCListbox (strict)"("ActiveCell"=w301, "CellBG"=w300, "ActiveCell"=w299, "CellBG"=w298) -> ()  [unwired: 2 in, 2 out]
            n133 = call <vilib>:"WPI_DashboardUpdate RPC Info.vi"("Operation"=w294) -> ("update"=w292:bool, "commands"=w291:string[][])  [unwired: 9 in]
            n134 = property on="Command Selection" class="MCListbox (strict)"("ItemNames"=w291) -> ()  [unwired: 2 in, 2 out]
            n135 = property on="Command Params" class="Tbl (strict)"("Active Cell"=w301, "Cell BG Color"=w300, "Active Cell"=w299, "Cell BG Color"=w298) -> ()  [unwired: 2 in, 2 out]
            n136 = call <vilib>:"WPI_DashboardUpdate Command Params.vi"("Update"=w292, "NewVal"=w293, "Commands"=w291, "Param Tbl"=w290) -> ()  [unwired: 7 in, 1 out]
          }
        }
        n137 = call <vilib>:"Connextion Info.vi"() -> ("Connected"=→"NT Connection":bool)  [unwired: 10 in, 1 out]
      }
      event "Test Tree": Value Change {
        # "Show appropriate\ncontrols"
        n138 = event-data() -> ("CtlRef"=w307:refnum<vi>, "NewVal"=w305:string)  [unwired: 1 in]
        n139 = call <vilib>:"WPI_UtilitiesGetTreeIOName.vi"("NewVal"=w305, "TreeControl in"=w307) -> ("I/O Name"=w308:string)  [unwired: 9 in]
        n140 = case shown="\"Camera\"" w308 {
          selector: w308 -> [_ w315 _ w337 w346 _]
          tunnel: w305 -> [_ _ w334 w336 _ w353]
          tunnel: cluster{string[]}[] [{["640x480", "320x240", "160x120"]}, {["Auto", "Fixed indoor", "Fixed outdoor 1", "Fixed outdoor 2", "Fixed fluorescent 1", "Fixed fluorescent 2", "Hold current"]}, {["Auto", "Flicker-free 50 Hz", "Flicker-free 60 Hz", "Hold current"]}, {["None", "Prioritize frame rate", "Prioritize image quality"]}, {["Monochrome", "Color"]}] -> [_ _ _ _ _ w352]
          frame Default {
            w310 = FALSE ("Visible")
            w309 = FALSE ("Visible")
            n141 = property on="Motor" class="Clust (strict)"("Visible"=w309) -> ()  [unwired: 2 in, 2 out]
            n142 = property on="Test Ring" class="Ring (strict)"("Visible"=w309) -> ()  [unwired: 2 in, 2 out]
            n143 = property on="Rev/Fwd" class="Clust (strict)"("Visible"=w310) -> ()  [unwired: 2 in, 2 out]
            n144 = property on="On/Off" class="Bool (strict)"("Visible"=w310) -> ()  [unwired: 2 in, 2 out]
            n145 = property on="Test Slider" class="Slide (strict)"("Visible"=w310) -> ()  [unwired: 2 in, 2 out]
          }
          frame "Analog Out", "Motor", "PWM" {
            w316 = FALSE ("Visible")
            n146 = case shown="\"Analog Out\"" w315 {
              tunnel: [1.0 ("Value") -1.0 ("Value") 0.0 ("Value")] -> w314
              tunnel: [255.0 ("Value") 1.0 ("Value") 5.0 ("Value")] -> w313
              tunnel: [128.0 ("Value") 0.0 ("Value") 0.0 ("Value")] -> w312
              tunnel: [64.0 ("Value") 0.5 ("Value") 1.0 ("Value")] -> w311
              frame "PWM" {
              }
              frame "Motor", Default {
              }
              frame "Analog Out" {
              }
            }
            n147 = property on="Motor" class="Clust (strict)"("Visible"=TRUE) -> ()  [unwired: 2 in, 2 out]
            n148 = property on="Value" class="Slide (strict)"("Value"=w312, "Scale.Minimum"=w314, "Scale.Maximum"=w313, "Scale.Increment"=w311) -> ()  [unwired: 2 in, 2 out]
            n149 = property on="On/Off" class="Bool (strict)"("Visible"=w316) -> ()  [unwired: 2 in, 2 out]
            n150 = property on="Test Slider" class="Slide (strict)"("Visible"=w316) -> ()  [unwired: 2 in, 2 out]
            n151 = property on="Test Ring" class="Ring (strict)"("Visible"=w316) -> ()  [unwired: 2 in, 2 out]
            n152 = property on="Rev/Fwd" class="Clust (strict)"("Visible"=w316) -> ()  [unwired: 2 in, 2 out]
          }
          frame "Servo" {
            w332 = FALSE ("Visible")
            n153 = call <vilib>:"NT Read Number.vi"("Name"=w334) -> ("Numeric"=w333:dbl)  [unwired: 9 in, 1 out]
            n154 = property on="Test Slider" class="Slide (strict)"("Visible"=TRUE, "Scale.Maximum"=170.0 ("Scale.Range:Maximum")) -> ()  [unwired: 2 in, 2 out]
            n155 = local write "Test Slider"(w333) -> ()
            n156 = property on="Motor" class="Clust (strict)"("Visible"=w332) -> ()  [unwired: 2 in, 2 out]
            n157 = property on="Rev/Fwd" class="Clust (strict)"("Visible"=w332) -> ()  [unwired: 2 in, 2 out]
            n158 = property on="On/Off" class="Bool (strict)"("Visible"=w332) -> ()  [unwired: 2 in, 2 out]
            n159 = property on="Test Ring" class="Ring (strict)"("Visible"=w332) -> ()  [unwired: 2 in, 2 out]
          }
          frame "Relay", "Solenoid" {
            w335 = FALSE ("Visible")
            n160 = property on="Motor" class="Clust (strict)"("Visible"=w335) -> ()  [unwired: 2 in, 2 out]
            n161 = property on="Test Slider" class="Slide (strict)"("Visible"=w335) -> ()  [unwired: 2 in, 2 out]
            n162 = Search and Replace String(input string=w336, search string="/Value  **", replace string="/Direction") -> (result string=w342:string)  [unwired: 5 in, 3 out]
            n163 = property on="Test Ring" class="Ring (strict)"("Visible"=w335) -> ()  [unwired: 2 in, 2 out]
            n164 = call <vilib>:"NT Read String.vi"("Name"=w342) -> ("String"=w340:string)  [unwired: 9 in, 1 out]
            n165 = Equal?(x="Both directions", y=w340) -> (x = y?=w338:bool)
            n166 = Not(x=w338) -> (.not. x?=w339:bool)
            n167 = property on="Rev/Fwd" class="Clust (strict)"("Visible"=w338) -> ()  [unwired: 2 in, 2 out]
            n168 = property on="On/Off" class="Bool (strict)"("Visible"=w339, "Caption.Text"=w337) -> ()  [unwired: 2 in, 2 out]
          }
          frame "Compressor", "Digital Out" {
            w345 = FALSE ("Visible")
            # "Get direction and finish"
            n169 = property on="Motor" class="Clust (strict)"("Visible"=w345) -> ()  [unwired: 2 in, 2 out]
            n170 = property on="Test Slider" class="Slide (strict)"("Visible"=w345) -> ()  [unwired: 2 in, 2 out]
            n171 = property on="Test Ring" class="Ring (strict)"("Visible"=w345) -> ()  [unwired: 2 in, 2 out]
            n172 = property on="On/Off" class="Bool (strict)"("Visible"=TRUE, "Caption.Text"=w346) -> ()  [unwired: 2 in, 2 out]
            n173 = property on="Rev/Fwd" class="Clust (strict)"("Visible"=FALSE) -> ()  [unwired: 2 in, 2 out]
          }
          frame "Camera" {
            n174 = call <vilib>:"Get Last Path Segment.vi"("String in"=w353) -> ("String out"=w354:string)  [unwired: 10 in]
            n175 = property on="On/Off" class="Bool (strict)"("Visible"=FALSE) -> ()  [unwired: 2 in, 2 out]
            n176 = property on="Motor" class="Clust (strict)"("Visible"=FALSE) -> ()  [unwired: 2 in, 2 out]
            n177 = property on="Rev/Fwd" class="Clust (strict)"("Visible"=FALSE) -> ()  [unwired: 2 in, 2 out]
            n178 = case shown="\"White Balance  **\"" w354 {
              tunnel: w353 -> [w360 w369 w378 w387 w396 _ w402]
              tunnel: w352 -> [w358 w366 w375 w384 w393 _ _]
              frame "Size  **" {
                n179 = Index Array(array=w358) -> (element=w357:cluster{string[]})  [unwired: 1 in]
                n180 = call <vilib>:"NT Read String.vi"("Name"=w360) -> ("String"=w359:string)  [unwired: 9 in, 1 out]
                n181 = Unbundle(w357) -> (w355:string[])
                n182 = Match First String(2:w355, 3:w359) -> (0:w356:i32)  [unwired: 1 out]
                n183 = property on="Test Ring" class="Ring (strict)"("Value"=w356, "Strings []"=w355) -> ()  [unwired: 2 in, 2 out]
                n184 = property on="Test Ring" class="Ring (strict)"("Visible"=TRUE) -> ()  [unwired: 2 in, 2 out]
                n185 = property on="Test Slider" class="Slide (strict)"("Visible"=FALSE) -> ()  [unwired: 2 in, 2 out]
              }
              frame "White Balance  **" {
                n186 = Index Array(array=w366, index=1) -> (element=w367:cluster{string[]})
                n187 = call <vilib>:"NT Read String.vi"("Name"=w369) -> ("String"=w368:string)  [unwired: 9 in, 1 out]
                n188 = Unbundle(w367) -> (w364:string[])
                n189 = Match First String(2:w364, 3:w368) -> (0:w363:i32)  [unwired: 1 out]
                n190 = property on="Test Ring" class="Ring (strict)"("Value"=w363, "Strings []"=w364) -> ()  [unwired: 2 in, 2 out]
                n191 = property on="Test Ring" class="Ring (strict)"("Visible"=TRUE) -> ()  [unwired: 2 in, 2 out]
                n192 = property on="Test Slider" class="Slide (strict)"("Visible"=FALSE) -> ()  [unwired: 2 in, 2 out]
              }
              frame "Exposure  **" {
                n193 = Index Array(array=w375, index=2) -> (element=w376:cluster{string[]})
                n194 = call <vilib>:"NT Read String.vi"("Name"=w378) -> ("String"=w377:string)  [unwired: 9 in, 1 out]
                n195 = Unbundle(w376) -> (w372:string[])
                n196 = Match First String(2:w372, 3:w377) -> (0:w373:i32)  [unwired: 1 out]
                n197 = property on="Test Ring" class="Ring (strict)"("Value"=w373, "Strings []"=w372) -> ()  [unwired: 2 in, 2 out]
                n198 = property on="Test Ring" class="Ring (strict)"("Visible"=TRUE) -> ()  [unwired: 2 in, 2 out]
                n199 = property on="Test Slider" class="Slide (strict)"("Visible"=FALSE) -> ()  [unwired: 2 in, 2 out]
              }
              frame "Exposure Priority  **" {
                n200 = Index Array(array=w384, index=3) -> (element=w385:cluster{string[]})
                n201 = call <vilib>:"NT Read String.vi"("Name"=w387) -> ("String"=w386:string)  [unwired: 9 in, 1 out]
                n202 = Unbundle(w385) -> (w381:string[])
                n203 = Match First String(2:w381, 3:w386) -> (0:w382:i32)  [unwired: 1 out]
                n204 = property on="Test Ring" class="Ring (strict)"("Value"=w382, "Strings []"=w381) -> ()  [unwired: 2 in, 2 out]
                n205 = property on="Test Ring" class="Ring (strict)"("Visible"=TRUE) -> ()  [unwired: 2 in, 2 out]
                n206 = property on="Test Slider" class="Slide (strict)"("Visible"=FALSE) -> ()  [unwired: 2 in, 2 out]
              }
              frame "Color Enable  **" {
                n207 = Index Array(array=w393, index=4) -> (element=w394:cluster{string[]})
                n208 = call <vilib>:"NT Read String.vi"("Name"=w396) -> ("String"=w395:string)  [unwired: 9 in, 1 out]
                n209 = Unbundle(w394) -> (w390:string[])
                n210 = Match First String(2:w390, 3:w395) -> (0:w391:i32)  [unwired: 1 out]
                n211 = property on="Test Ring" class="Ring (strict)"("Value"=w391, "Strings []"=w390) -> ()  [unwired: 2 in, 2 out]
                n212 = property on="Test Ring" class="Ring (strict)"("Visible"=TRUE) -> ()  [unwired: 2 in, 2 out]
                n213 = property on="Test Slider" class="Slide (strict)"("Visible"=FALSE) -> ()  [unwired: 2 in, 2 out]
              }
              frame Default {
                n214 = property on="Test Ring" class="Ring (strict)"("Visible"=FALSE) -> ()  [unwired: 2 in, 2 out]
                n215 = property on="Test Slider" class="Slide (strict)"("Visible"=FALSE) -> ()  [unwired: 2 in, 2 out]
              }
              frame "Brightness  **", "Color Level  **", "Compression  **", "FPS  **", "Sharpness  **" {
                n216 = call <vilib>:"NT Read Number.vi"("Name"=w402) -> ("Numeric"=w401:dbl)  [unwired: 9 in, 1 out]
                n217 = local write "Test Slider"(w401) -> ()
                n218 = property on="Test Slider" class="Slide (strict)"("Visible"=TRUE, "Scale.Maximum"=100.0 ("Scale.Range:Maximum")) -> ()  [unwired: 2 in, 2 out]
                n219 = property on="Test Ring" class="Ring (strict)"("Visible"=FALSE) -> ()  [unwired: 2 in, 2 out]
              }
            }
          }
        }
        n220 = property on="Progress" class="Clust (strict)"("Visible"=FALSE) -> ()  [unwired: 2 in, 2 out]
      }
      event "Test Name": Mouse Enter {
        # "Populate the ring with the list of tests"
        n221 = event-data() -> ()  [unwired: 1 in, 1 out]
        n222 = call <vilib>:"NT Read String Array.vi"("Name"="TestMode/TestList") -> ("String Array"=w410:string[])  [unwired: 9 in, 1 out]
        n223 = Build Array (concatenate)("Select the test to run...", w410) -> (w409:string[])
        n224 = property on="Test Name" class="Ring (strict)"("Strings []"=w409) -> ()  [unwired: 2 in, 2 out]
      }
      event "Test Name": Value Change {
        w412 = FALSE ("Visible")
        # "Tell the robot the test name to run"
        n225 = event-data() -> ("NewVal"=w416:u16)  [unwired: 1 in]
        n226 = property on="Test Name" class="Ring (strict)"() -> ("Strings []"=w417:string[])  [unwired: 2 in, 2 out]
        n227 = local write "Progress"(T6 {"Test Progress"=0, "Test Progress Text"=""} ("Progress")) -> ()
        n228 = Index Array(array=w417, index=w416) -> (element=w415:string)
        n229 = call <vilib>:"NT Write String.vi"("String"=w415, "Name"="TestMode/TestName") -> ()  [unwired: 9 in, 1 out]
        n230 = property on="Progress" class="Clust (strict)"("Visible"=TRUE) -> ()  [unwired: 2 in, 2 out]
        n231 = property on="Motor" class="Clust (strict)"("Visible"=w412) -> ()  [unwired: 2 in, 2 out]
        n232 = property on="Test Slider" class="Slide (strict)"("Visible"=w412) -> ()  [unwired: 2 in, 2 out]
        n233 = property on="On/Off" class="Bool (strict)"("Visible"=w412) -> ()  [unwired: 2 in, 2 out]
        n234 = property on="Rev/Fwd" class="Clust (strict)"("Visible"=w412) -> ()  [unwired: 2 in, 2 out]
        n235 = property on="Test Ring" class="Ring (strict)"("Visible"=w412) -> ()  [unwired: 2 in, 2 out]
      }
      event "Select Auto": Mouse Enter {
        # "Populate the combo box with the list of autonomous options"
        n236 = event-data() -> ()  [unwired: 1 in, 1 out]
        n237 = call <vilib>:"NT Read String Array.vi"("Name"="Auto List") -> ("String Array"=w419:string[])  [unwired: 9 in, 1 out]
        n238 = property on="Select Auto" class="CmbBox"("Strings[]"=w419) -> ()  [unwired: 2 in, 2 out]
      }
      event "Select Auto": Value Change {
        # "User modified the Auto Selection. Write to NT variable so robot knows."
        n239 = event-data() -> ("NewVal"=w422:string)  [unwired: 1 in]
        n240 = call <vilib>:"NT Write String.vi"("String"=w422, "Name"="Auto Selector") -> ()  [unwired: 9 in, 1 out]
      }
      event "Command Selection": Value Change {
        # "Get the params and show in table"
        n241 = event-data() -> ("NewVal"=w428:i32)  [unwired: 1 in]
        n242 = property on="Command Selection" class="MCListbox (strict)"() -> ("ItemNames"=w426:string[][])  [unwired: 2 in, 2 out]
        n243 = call <vilib>:"WPI_DashboardUpdate Command Params.vi"("NewVal"=w428, "Commands"=w426, "Param Tbl"=w427) -> ()  [unwired: 8 in, 1 out]
      }
      event "Execute Command": Value Change {
        # "Started one, Unique ID holds\nresponse"
        n244 = event-data() -> ()  [unwired: 1 in, 1 out]
        n245 = property on="Command Selection" class="MCListbox (strict)"() -> ("ItemNames"=w439:string[][])  [unwired: 2 in, 2 out]
        n246 = Index Array(array=w439, index (row)="Command Selection", index (col)=0) -> (element=w437:string)
        n247 = call <vilib>:"Invoke Commands.vi"("Command Params"="Command Params", "Function Name"=w437) -> ("Params"=w433:u8, "Started"=w432:bool)  [unwired: 7 in, 1 out]
        n248 = Array Subset(array="Command Params", length (row)=w433) -> (w434:string[][])  [unwired: 3 in]
        n249 = Select(t="Executing" ("Cmd Status"), s=w432, f="" ("Cmd Status")) -> (s? t:f=→"Cmd Status":string)
      }
      event "Command Selection": Double Click {
        n250 = event-data() -> ("Row"=w447:i32)  [unwired: 1 in]
        n251 = property on="Command Selection" class="MCListbox (strict)"() -> ("ItemNames"=w450:string[][])  [unwired: 2 in, 2 out]
        n252 = local read "Command Params"() -> (w446:string[][])
        n253 = Index Array(array=w450, index (row)=w447, index (col)=0) -> (element=w448:string)
        n254 = call <vilib>:"Invoke Commands.vi"("Command Params"=w446, "Function Name"=w448) -> ("Params"=w445:u8, "Started"=w440:bool)  [unwired: 7 in, 1 out]
        n255 = Array Subset(array=w446, length (row)=w445) -> (w444:string[][])  [unwired: 3 in]
        n256 = Select(t="Executing" ("Cmd Status"), s=w440, f="" ("Cmd Status")) -> (s? t:f=w441:string)
        n257 = local write "Cmd Status"(w441) -> ()
      }
      event "CheckList": Double Click {
        # "Shift clears all"
        # "Update symbols on the listbox"
        n258 = event-data() -> ("PlatMods.Shift"=w452:bool, "Row"=w454:i32)  [unwired: 1 in]
        n259 = case shown="True" w452 {
          tunnel: w454 -> [w458 _]
          tunnel: 1 -> [w457 _]
          frame False {
            n260 = property on="CheckList" class="LstBox (strict)"() -> ("Item Symbols"=w456:i32[])  [unwired: 2 in, 2 out]
            n261 = Replace Array Subset(array=w456, new element=w457, index=w458) -> (w455:i32[])
            n262 = property on="CheckList" class="LstBox (strict)"("Item Symbols"=w455) -> ()  [unwired: 2 in, 2 out]
          }
          frame True {
            w459 = 0 ("Top Row")
            n263 = property on="CheckList" class="LstBox (strict)"() -> ("Number of Rows"=w461:u32)  [unwired: 2 in, 2 out]
            n264 = Initialize Array(0, w461) -> (w460:i32[])
            n265 = property on="CheckList" class="LstBox (strict)"("Top Row"=w459, "Value"=w459, "Item Symbols"=w460) -> ()  [unwired: 2 in, 2 out]
          }
        }
      }
      event "CheckList": Key Down {
        # "Update symbols on the listbox\nLeft and right keys check and uncheck"
        n266 = event-data() -> ("VKey"=w465:T21)  [unwired: 1 in]
        n267 = case shown="\"Left\", \"Right\"" w465 {
          selector: w465 -> [w470 _]
          tunnel: eventvkey."Left" ("VKey") -> [w468 _]
          frame "Left", "Right" {
            n268 = Equal?(x=w468, y=w470) -> (x = y?=w469:bool)
            n269 = Select(t=0, s=w469, f=1) -> (s? t:f=w471:i32)
            n270 = property on="CheckList" class="LstBox (strict)"() -> ("Item Symbols"=w474:i32[])  [unwired: 2 in, 2 out]
            n271 = Replace Array Subset(array=w474, new element=w471, index="CheckList") -> (w473:i32[])
            n272 = property on="CheckList" class="LstBox (strict)"("Item Symbols"=w473) -> ()  [unwired: 2 in, 2 out]
          }
          frame Default {
          }
        }
      }
      event "Motor.Enable": Value Change {
        # "When the test mode otor enable helper is set, update that\ntree row item's value"
        n273 = event-data() -> ("NewVal"=w480:bool)  [unwired: 1 in]
        n274 = Unbundle("Motor") -> ("Value"=w479:dbl)  [unwired: 1 out]
        n275 = Select(t=w479, s=w480, f=0.0) -> (s? t:f=w477:dbl)
        n276 = call <vilib>:"NT Write Number.vi"("Numeric"=w477, "Name"=w476) -> ()  [unwired: 9 in, 1 out]
      }
      event "Test Slider": Value Change {
        # "When the test mode slider helper is set, update that\ntree row item's value"
        n277 = event-data() -> ("NewVal"=w483:dbl)  [unwired: 1 in]
        n278 = call <vilib>:"NT Write Number.vi"("Numeric"=w483, "Name"=w484) -> ()  [unwired: 9 in, 1 out]
      }
      event "On/Off": Value Change {
        # "When the test mode on/off helper value is set, update that\ntree row item's value"
        n279 = event-data() -> ("NewVal"=w488:bool)  [unwired: 1 in]
        n280 = Boolean To (0,1)(Boolean=w488) -> (0, 1=w487:i16)
        n281 = call <vilib>:"NT Write Number.vi"("Numeric"=w487, "Name"=w486) -> ()  [unwired: 9 in, 1 out]
      }
      event "Rev/Fwd": Value Change {
        # "When the test mode helper value for relays is set, update that\ntree row item's value"
        n282 = event-data() -> ("NewVal.Forward"=w496:bool, "NewVal.Reverse"=w495:bool)  [unwired: 1 in]
        n283 = Boolean To (0,1)(Boolean=w496) -> (0, 1=w492:i16)
        n284 = Boolean To (0,1)(Boolean=w495) -> (0, 1=w494:i16)
        n285 = Negate(x=w494) -> (-x=w493:i16)
        n286 = Add(x=w492, y=w493) -> (x+y=w491:i16)
        n287 = call <vilib>:"NT Write Number.vi"("Numeric"=w491, "Name"=w490) -> ()  [unwired: 9 in, 1 out]
      }
      event "Test Ring": Value Change {
        # "When a test mode helper value is selected from the ring,\nset the tree item's variable to the string value"
        n288 = event-data() -> ("NewVal"=w500:u16)  [unwired: 1 in]
        n289 = property on="Test Ring" class="Ring (strict)"() -> ("Strings []"=w501:string[])  [unwired: 2 in, 2 out]
        n290 = Index Array(array=w501, index=w500) -> (element=w499:string)
        n291 = call <vilib>:"NT Write String.vi"("String"=w499, "Name"=w498) -> ()  [unwired: 9 in, 1 out]
      }
      event "Rec Mode": Value Change {
        # "Update globals for recording mode and path to read log from.\nClear when logging and let NetworkTables set path for vision to\nuse."
        n292 = event-data() -> ("NewVal"=w512:enum32{"Stop", "Record", "Playback"})  [unwired: 1 in]
        n293 = global write "WPI_DashboardLogging Global.vi" "Logging Filename"(path "") -> ()
        n294 = global write "WPI_DashboardLogging Global.vi" "Recording"(w512) -> ()
        n295 = case shown="\"Playback\"" w512 {
          tunnel: w511 -> [_ w514 w523]
          tunnel: [_ _ w522] -> w509
          tunnel: [_ _ w521] -> _
          tunnel: w507 -> [_ _ w519]
          tunnel: cluster{i32, i32} {-250, 170} -> [_ _ w518]
          tunnel: [_ _ T22 {"Image Size"=TRUE, "Image Type"=TRUE, "Pixel Value"=TRUE, "ROI Information"=TRUE, "Zoom Factor"=FALSE} ("Image Information Shown:All Elements")] -> w502
          tunnel: [_ _ TRUE ("Zoom Factor")] -> w503
          tunnel: w505 -> [_ _ w515]
          frame Default {
          }
          frame "Stop", "Record" {
            # "Place Window too"
            n296 = invoke class="VI" method="FP.Close"(reference=w514) -> (reference out=w513:refnum<vi>)  [unwired: 2 in, 2 out]
            n297 = invoke class="VI" method="Abort VI"(reference=w513) -> ()  [unwired: 2 in, 3 out]
          }
          frame "Playback" {
            n298 = call "Open Playback Panel.vi"("Offset"=w518, "DB VI Ref"=w519, "Playback in"=w523) -> ("Playback out"=w520:refnum<vi>)  [unwired: 8 in]
            n299 = register-events(w520, w515) -> (reference out=w522:refnum<event-registration>, error out=w521:errorcluster)  [unwired: 2 in]
          }
        }
        n300 = property on="Camera Image Right" class="ImageControl"("Image Information Shown"=w502, "Image Information Visible"=w503) -> ()  [unwired: 2 in, 2 out]
        n301 = property on="Camera Image" class="ImageControl"("Image Information Shown"=w502, "Image Information Visible"=w503) -> ()  [unwired: 2 in, 2 out]
        n302 = call <vilib>:"WPI_DashboardNT Log FieldName Cache.vi"("Operation"=enum16{"Lookup/Add", "Index", "Clear"}."Clear") -> ()  [unwired: 8 in, 3 out]
      }
      event Panel Close {
        w525 = enum32{"Stop", "Record", "Playback"}."Stop" ("Rec Mode")
        # "Playback window has been closed, abort"
        n303 = event-data() -> ()  [unwired: 1 in, 4 out]
        n304 = local write "Rec Mode"(w525) -> ()
        n305 = global write "WPI_DashboardLogging Global.vi" "Recording"(w525) -> ()
      }
      event Panel Close {
        # "Abort playback window and ourself"
        n306 = event-data() -> ()  [unwired: 1 in, 4 out]
        n307 = invoke class="VI" method="FP.Close"(reference=w529) -> (reference out=w528:refnum<vi>)  [unwired: 2 in, 2 out]
        n308 = invoke class="VI" method="Abort VI"(reference=w528) -> (error out=w527:errorcluster)  [unwired: 2 in, 2 out]
        n309 = invoke class="VI" method="Abort VI"(error in=w527) -> ()  [unwired: 2 in, 3 out]
      }
      event User Event {
        n310 = event-data() -> ("IDs"=w536:cluster{"RPC field ID":u16, "Unique ID":u16}, "String"=w535:string)  [unwired: 1 in]
        n311 = Bundle("IDs"=w536, "String"=w535) -> (w534:T9)  [unwired: 1 in]
        n312 = call <vilib>:"Retrieve RPC Response.vi"("RPC Response"=w534) -> ("Output"=w532:string[][])  [unwired: 10 in]
        n313 = Build Array (concatenate)(w530, w532) -> (w531:string[][])
        n314 = local write "Command Params"(w531) -> ()
        n315 = local write "Cmd Status"("" ("Cmd Status")) -> ()
      }
      event "Tree": Double Click {
        n316 = event-data() -> ("PlatMods"=w542:T25, "Tag"=w539:string)  [unwired: 1 in]
        n317 = Unbundle(w542) -> ("Shift"=w541:bool)  [unwired: 4 out]
        n318 = String Subset(string=w539, length (rest)=1 ("length (rest)")) -> (substring=w538:string)  [unwired: 1 in]
        n319 = Not(x=w541) -> (.not. x?=w540:bool)
        n320 = case shown="\"/\"" w538 {
          tunnel: w539 -> [_ w545]
          tunnel: w540 -> [_ w544]
          frame Default {
          }
          frame "/" {
            n321 = call <vilib>:"NT Update Persistence.vi"("Persistence"=w544, "Name"=w545) -> ()  [unwired: 9 in, 1 out]
          }
        }
      }
    }
  }
  n322 = while {
    tunnel: w111 -> [w547]
    i -> [w550]
    stop <- FALSE stop-if-true
    n323 = Wait (ms)(milliseconds to wait=u32 100) -> ()  [unwired: 1 out]
    n324 = case shown="\"Playback\"" "Rec Mode" {
      tunnel: w550 -> [_ _ w565]
      tunnel: [u32 2829099 ("Base Color") u32 11141120 ("Target Color") w554] -> w546
      frame "Stop", Default {
        # "Reset the color, extra updates don't cost much"
      }
      frame "Record" {
      }
      frame "Playback" {
        # "Playback"
        n325 = Quotient & Remainder(x=w565, y=u32 50 ("milliseconds to wait")) -> (x-y*floor(x/y)=w561:u32)  [unwired: 1 out]
        n326 = Divide(x=w561, y=u32 50 ("milliseconds to wait")) -> (x/y=w558:dbl)
        n327 = Multiply(x=6.283185307179586, y=w558) -> (x*y=w563:dbl)
        n328 = Sine(x=w563) -> (sin(x)=w562:dbl)
        n329 = Absolute Value(x=w562) -> (abs(x)=w555:dbl)
        n330 = call "Interpolate RGB Color.vi"("Proportion"=w555, "Target Color"=u32 30976, "Base Color"=u32 2829099) -> ("Result Color"=w554:u32)  [unwired: 8 in]
      }
    }
    n331 = property class="Pane"(reference=w547, "PaneColor"=w546) -> ()  [unwired: 1 in, 2 out]
  }
  n332 = local write "Dashboard Tab"(T2."Drive" ("Dashboard Tab")) -> ()
  n333 = property on="On/Off" class="Bool (strict)"("Visible"=w82) -> ()  [unwired: 2 in, 2 out]
  n334 = property on="Motor" class="Clust (strict)"("Visible"=w82) -> ()  [unwired: 2 in, 2 out]
  n335 = property on="Progress" class="Clust (strict)"("Visible"=w82) -> ()  [unwired: 2 in, 2 out]
  n336 = property on="Test Ring" class="Ring (strict)"("Visible"=w82) -> ()  [unwired: 2 in, 2 out]
  n337 = property on="Rev/Fwd" class="Clust (strict)"("Visible"=w82) -> ()  [unwired: 2 in, 2 out]
  n338 = while {
    tunnel: u16 1741 ("timeout ms (25000)") -> [w567]
    stop <- FALSE stop-if-true
    n339 = TCP Create Listener(10:w567) -> (0:w566:errorcluster, 3:w568:refnum<k5>)  [unwired: 4 in, 1 out]
    n340 = case shown="No Error" w566 {
      selector: w566 -> [w570 _]
      tunnel: w568 -> [w571 _]
      frame No Error {
        n341 = while {
          tunnel: w571 -> [w574]
          tunnel: w570 -> [w573]
          stop <- FALSE stop-if-true
          n342 = TCP Wait On Listener(8:w573, 11:w574) -> (0:w575:errorcluster, 4:w576:refnum<k5>)  [unwired: 2 in, 3 out]
          n343 = local write "TCP"(w576) -> ()
          n344 = case shown="No Error" w575 {
            frame No Error {
            }
            frame Error {
              n345 = Wait (ms)(milliseconds to wait=u32 1000) -> ()  [unwired: 1 out]
            }
          }
        }
      }
      frame Error {
        n346 = Wait (ms)(milliseconds to wait=u32 1000) -> ()  [unwired: 1 out]
      }
    }
  }
  n347 = local write "Command Selection"(u16 0 ("milliseconds to wait")) -> ()
  n348 = local write "Command Params"(string[][] [] ("Command Params")) -> ()
  n349 = global write "WPI_DashboardLogging Global.vi" "Recording"(w105) -> ()
  n350 = local write "Rec Mode"(w105) -> ()
  n351 = call <vilib>:"WPI_DriverStationGame Specific Data.vi"() -> ("Game Specific Data"=w4:string)  [unwired: 11 in]
  n352 = call <vilib>:"NT Write String.vi"("String"="Select Auto", "Name"="Auto Selector") -> ()  [unwired: 9 in, 1 out]
  n353 = String Subset(string=w4, offset (0)=1, length (rest)=1 ("length (rest)")) -> (substring=w28:string)
  n354 = String Subset(string=w4, offset (0)=0, length (rest)=1 ("length (rest)")) -> (substring=w44:string)
  n355 = String Subset(string=w4, offset (0)=2, length (rest)=1 ("length (rest)")) -> (substring=w16:string)
  n356 = Equal?(x=w28, y="\"L\"") -> (x = y?=w24:bool)
  n357 = Equal?(x=w44, y="\"L\"") -> (x = y?=w38:bool)
  n358 = Equal?(x=w16, y="\"L\"") -> (x = y?=w12:bool)
  n359 = Equal?(x="What color are you?", y="\"Red\"") -> (x = y?=w1:bool)
  n360 = Not(x=w24) -> (.not. x?=w25:bool)
  n361 = Not(x=w38) -> (.not. x?=w39:bool)
  n362 = Not(x=w12) -> (.not. x?=w13:bool)
  n363 = Select(t=w25, s=w1, f=w24) -> (s? t:f=w21:bool)
  n364 = Select(t=w39, s=w1, f=w38) -> (s? t:f=w34:bool)
  n365 = Select(t=w13, s=w1, f=w12) -> (s? t:f=w9:bool)
  n366 = Select(t=u32 16860 ("L1"), s=w21, f=u32 16711680 ("L1")) -> (s? t:f=→"L2":u32)
  n367 = Select(t=u32 16860 ("L1"), s=w34, f=u32 16711680 ("L1")) -> (s? t:f=→"L1":u32)
  n368 = Select(t=u32 16860 ("L1"), s=w9, f=u32 16711680 ("L1")) -> (s? t:f=→"L3":u32)
  n369 = Not(x=w21) -> (.not. x?=w20:bool)
  n370 = Not(x=w34) -> (.not. x?=w33:bool)
  n371 = Not(x=w9) -> (.not. x?=w8:bool)
  n372 = Select(t=u32 16860 ("L1"), s=w20, f=u32 16711680 ("L1")) -> (s? t:f=→"R2":u32)
  n373 = Select(t=u32 16860 ("L1"), s=w33, f=u32 16711680 ("L1")) -> (s? t:f=→"R1":u32)
  n374 = Select(t=u32 16860 ("L1"), s=w8, f=u32 16711680 ("L1")) -> (s? t:f=→"R3":u32)
